vi "RoundToHalf.vi"(11 "Cluster in":T1) -> (3 "Cluster out":T1)   [LabVIEW 2014, in "Manipulator.lvclass"]
uses:
  Manipulator.lvclass
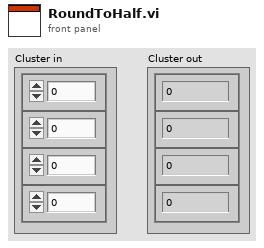
[diagram p1: front panel]
types:
  T1 = cluster{"Numeric Control":dbl, "Numeric Control":dbl, "Numeric Control":dbl, "Numeric Control":dbl}
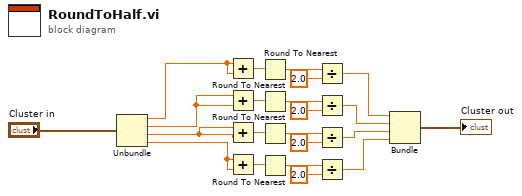
[diagram p0: block diagram]
diagram:
  n1 = Unbundle("Cluster in") -> ("Numeric Control"=w17:dbl, "Numeric Control"=w18:dbl, "Numeric Control"=w21:dbl, "Numeric Control"=w22:dbl)
  n2 = Add(x=w17, y=w17) -> (x+y=w3:dbl)
  n3 = Add(x=w18, y=w18) -> (x+y=w5:dbl)
  n4 = Add(x=w21, y=w21) -> (x+y=w11:dbl)
  n5 = Add(x=w22, y=w22) -> (x+y=w13:dbl)
  n6 = Round To Nearest(number=w3) -> (nearest integer value=w2:dbl)
  n7 = Round To Nearest(number=w5) -> (nearest integer value=w6:dbl)
  n8 = Round To Nearest(number=w11) -> (nearest integer value=w10:dbl)
  n9 = Round To Nearest(number=w13) -> (nearest integer value=w14:dbl)
  n10 = Divide(x=w2, y=2.0) -> (x/y=w4:dbl)
  n11 = Divide(x=w6, y=2.0) -> (x/y=w8:dbl)
  n12 = Divide(x=w10, y=2.0) -> (x/y=w12:dbl)
  n13 = Divide(x=w14, y=2.0) -> (x/y=w16:dbl)
  n14 = Bundle(w4, w8, w12, w16) -> (→"Cluster out":cluster{dbl, dbl, dbl, dbl})  [unwired: 1 in]
